vi "PXI_Host_SGL_Read_OldMethod_Benchmark.vi"() -> ()   [LabVIEW 2018]
uses:
  <vilib>/Platform/TimedLoop/XDataNode/timing_clust.ctl
  <vilib>/Platform/TimedLoop/XDataNode/nitl_modes.ctl
  <vilib>/Platform/TimedLoop/XDataNode/wakeup.ctl
  <vilib>/addons/FPGA Advanced Session Resources/LVFPGA Adv Session Resources/OpenByNameSubVI.vi
  <vilib>/rvi/interface/common/dynamic/niFpgaEscapeDelimiterAndNull.vi
  <vilib>/Utility/error.llb/Error Cluster From Error Code.vi
  <vilib>/rvi/errors/niLvFpgaAdjustHostInterfaceError.vi
  <vilib>/FPGAPlugInAG/Dynamic/niLvFpga_Close_Dynamic.vi
  <vilib>/addons/FPGA Advanced Session Resources/LVFPGA Adv Session Resources/OpenByName.xnode
  <vilib>/platform/TimedLoop/XDataNode/XDataNode.xnode
  <vilib>/rvi/interface/nirviReadWriteControl/nirviReadWriteControl.xnode
  <vilib>/rvi/interface/nirviCloseFPGA/nirviCloseFPGA.xnode
  NiFpgaLv.dll
  <vilib>/rvi/interface/Simulation/niFpgaSimulationCallBeginRW.vi
  <vilib>/Platform/TimedLoop/XDataNode/XDNodeRunTimeDep.lvlib
  <vilib>/addons/FPGA Advanced Session Resources/LVFPGA Adv Session Resources/LVFPGAAdvSessionResources.lvlib
panel:
  out "Waveform Graph":dbl[](graph)
  out "Standard Dev":dbl
  out "Execution time (s)":dbl
  out "Maximum(s)":dbl
  out "Value out":sgl
  out "error out":errorcluster
  # "Recorded time"
  # "3.37551E-5"
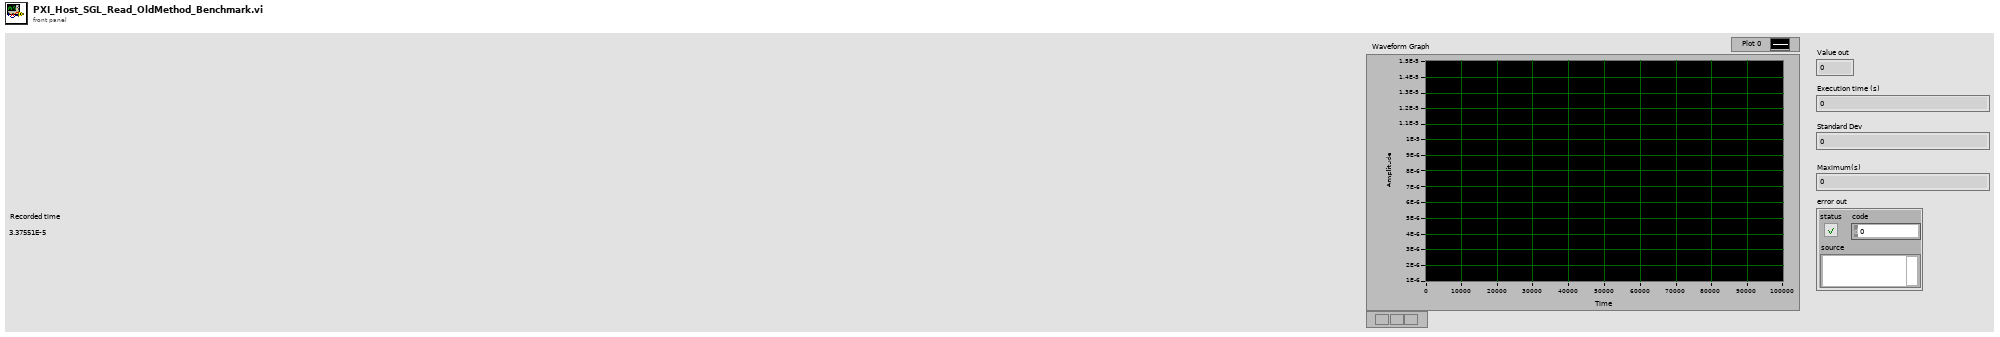
[diagram p1: front panel]
types:
  T1 = typedef "XDNodeRunTimeDep.lvlib/timing_clust.ctl" = cluster{"Expected End [f-1]":u64, "Actual End [f-1]":u64, "Finished Late? [f-1]":bool, "Expected End [i-1]":u64, "Actual End [i-1]":u64, "Finished Late? [i-1]":bool, "Expected Start [i]":u64, "Actual Start [i]":u64, "Expected Start [f]":u64, "Actual Start [f]":u64, "Source Name":string, "Structure Name":string, "Period":i64, "Deadline":i64, "Offset":i64, "Start":i64, "Priority":i32, "Timeout":i32, "Mode":T2, "Wakeup Reason":T3, "Error":errorcluster, "Source Type":string, "Secondary Source Type":string, "Global End Time":u64, "Global Start Time":u64, "Frame Duration":u64, "Iteration Duration":u64, "Assigned CPU":i32, "I/O Scan Engine Mode":u32}
  T2 = typedef "XDNodeRunTimeDep.lvlib/nitl_modes.ctl" = enum32{"No Change", "Process missed periods, maintain original phase", "Discard missed periods, maintain original phase", "Process missed periods, ignore original phase", "Discard missed periods, ignore original phase"}
  T3 = typedef "XDNodeRunTimeDep.lvlib/wakeup.ctl" = enum32{"Normal", "Aborted", "Asynchronous wakeup", "Timing source error", "Timed loop error", "Timeout"}
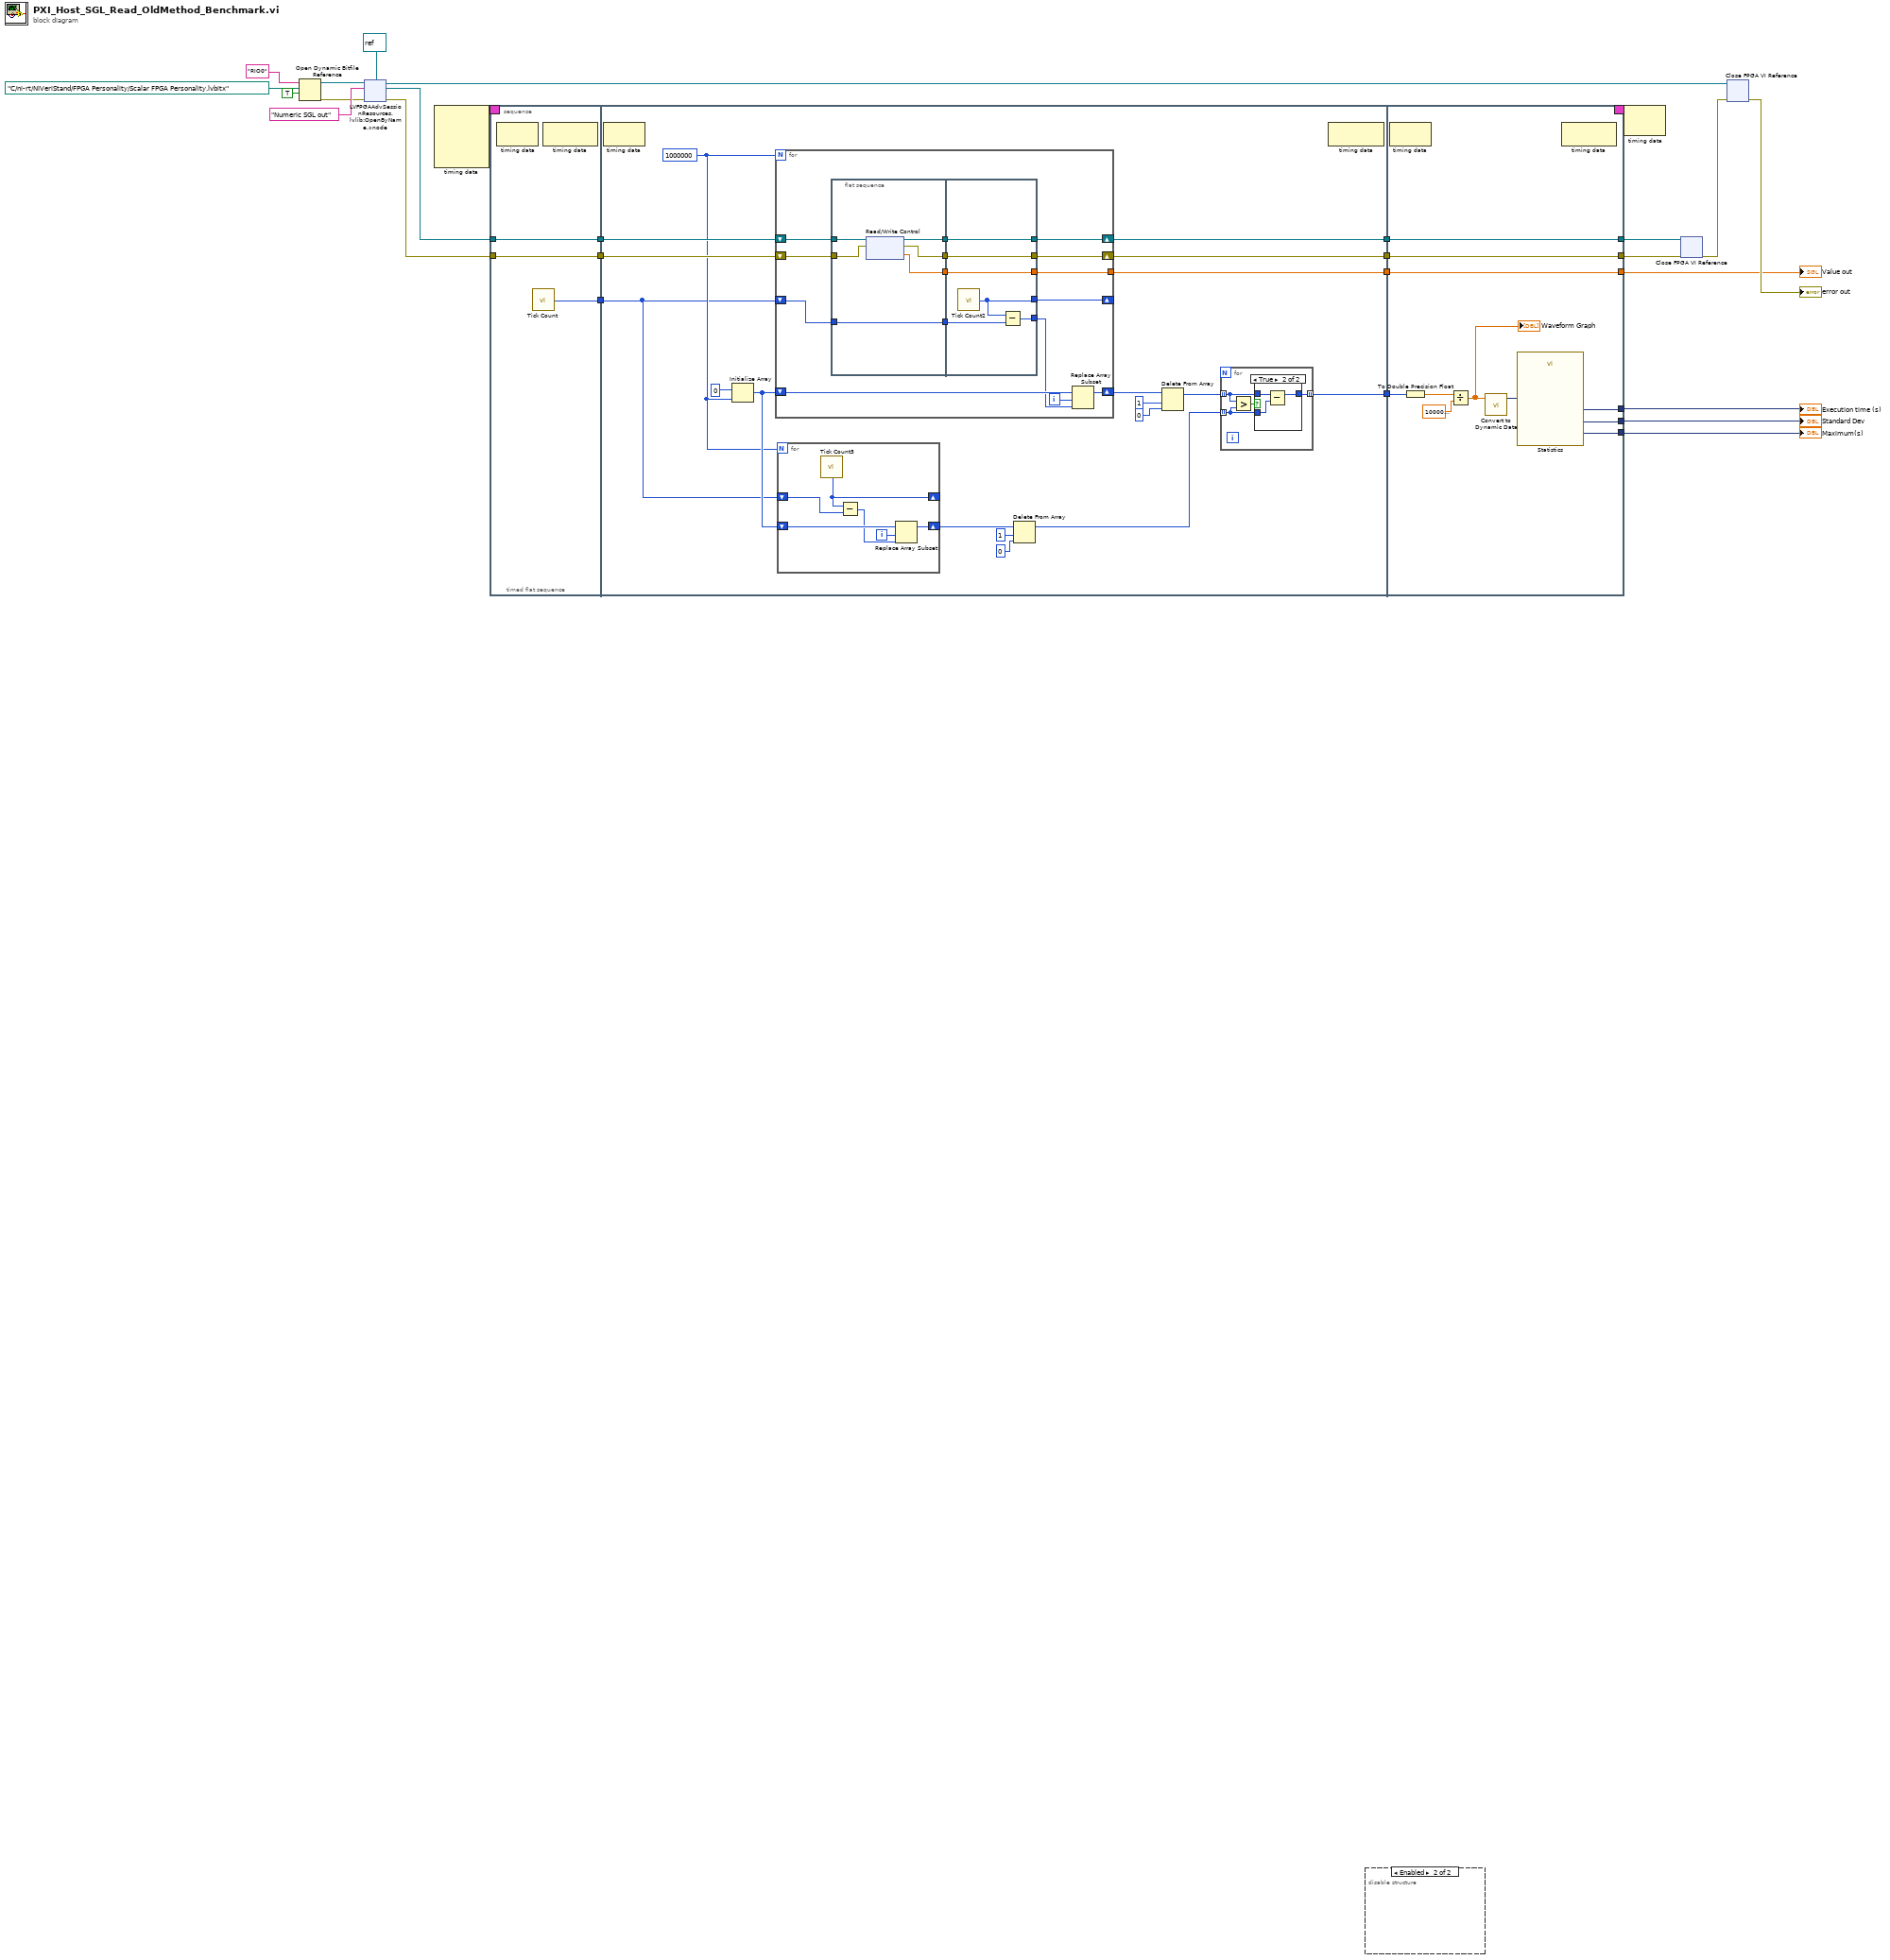
[diagram p0: block diagram]
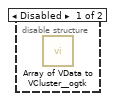
[diagram p3: hidden frame]
diagram:
  n1 = Open Dynamic Bitfile Reference(0:"RIO0" ("Device address"), 1:path "C:/ni-rt/NIVeriStand/FPGA Personality/Scalar FPGA Personality.lvbitx" ("Bitfile path"), 2:TRUE ("Run When Loaded")) -> (5:w16:refnum<k20>, 8:w14:errorcluster)  [unwired: 2 in]
  n2 = xnode "LVFPGAAdvSessionResources.lvlib:OpenByName.xnode"("FPGA VI Reference in"=w16, "Resource name in"="Numeric SGL out", "Single resource reference type in"=refnum<k20> refnum ("Type"), "Error in"=w14) -> ("Single resource reference out"=w12:refnum<k20>, "Error out"=w13:errorcluster, "FPGA VI Reference out"=w8:refnum<k20>)
  n3 = node-c288() -> (w5:T1)  [unwired: 4 in]
  n4 = timed-sequence {
    timing: w5 -> [_]
    timing-out: [_] -> w4
    tunnel: [w35] -> w17
    tunnel: w13 -> [w34]
    tunnel: w12 -> [w33]
    tunnel: [w32] -> w10
    tunnel: [w31] -> w6
    tunnel: [w23] -> w3
    tunnel: [w22] -> w2
    tunnel: [w21] -> w1
    n5 = timed-flat-sequence {
      tunnel: w33 -> [w37]
      tunnel: w34 -> [w38]
      tunnel: [w38] -> w30
      tunnel: [w37] -> w29
      tunnel: [w36] -> w28
      tunnel: w30 -> [w57]
      tunnel: w29 -> [w56]
      tunnel: w28 -> [w41]
      tunnel: [w58] -> w27
      tunnel: [w55] -> w26
      tunnel: [w54] -> w25
      tunnel: [w42] -> w24
      tunnel: [w110] -> w31
      tunnel: [w111] -> w32
      tunnel: [w112] -> w35
      tunnel: w27 -> [w112]
      tunnel: w26 -> [w111]
      tunnel: w25 -> [w110]
      tunnel: w24 -> [w105]
      tunnel: [w104] -> w23
      tunnel: [w103] -> w22
      tunnel: [w102] -> w21
      frame #0 {
        n6 = node-c288() -> ()  [unwired: 1 in, 1 out]
        n7 = call "Tick Count"() -> ("Tick Count(Ticks)"=w36:u32)
        n8 = node-c288() -> ()  [unwired: 1 in, 1 out]
      }
      frame #1 {
        w43 = 1000000
        n9 = node-c288() -> ()  [unwired: 1 in, 1 out]
        n10 = Initialize Array(u32 0 ("Tick Count(uSec)"), w43) -> (w44:u32[])
        n11 = for {
          N: w43 -> [_]
          tunnel: [w76] -> w54
          shift-right: [w80] -> w58
          shift-left: w57 -> [w79]
          shift-right: [w77] -> w55
          shift-left: w56 -> [w78]
          shift-right: [w73] -> _
          shift-left: w41 -> [w75]
          shift-right: [w69] -> w46
          shift-left: w44 -> [w72]
          i -> [w70]
          n12 = flat-sequence {
            tunnel: [w87] -> w83
            tunnel: [w86] -> w82
            tunnel: [w85] -> w81
            tunnel: w78 -> [w89]
            tunnel: w79 -> [w88]
            tunnel: w75 -> [w84]
            tunnel: [w84] -> w74
            tunnel: [w95] -> w71
            tunnel: w83 -> [w94]
            tunnel: [w94] -> w80
            tunnel: [w93] -> w76
            tunnel: w82 -> [w93]
            tunnel: w81 -> [w92]
            tunnel: [w92] -> w77
            tunnel: w74 -> [w91]
            tunnel: [w90] -> w73
            frame #0 {
              n13 = xnode "Read/Write Control"("FPGA VI Reference In"=w89, "error in"=w88) -> ("FPGA VI Reference Out"=w85:refnum<k20>, "error out"=w87:errorcluster, "Value"=w86:sgl)
            }
            frame #1 {
              n14 = call "Tick Count2"() -> ("Tick Count(Ticks)"=w90:u32)
              n15 = Subtract(x=w90, y=w91) -> (x-y=w95:u32)
            }
          }
          n16 = Replace Array Subset(array=w72, new element=w71, index=w70) -> (w69:u32[])
        }
        n17 = for {
          N: w43 -> [_]
          shift-right: [w96] -> w50
          shift-left: w44 -> [w99]
          shift-right: [w101] -> _
          shift-left: w41 -> [w100]
          i -> [w97]
          n18 = call "Tick Count3"() -> ("Tick Count(Ticks)"=w101:u32)
          n19 = Subtract(x=w101, y=w100) -> (x-y=w98:u32)
          n20 = Replace Array Subset(array=w99, new element=w98, index=w97) -> (w96:u32[])
        }
        n21 = Delete From Array(array=w50, length=1, index=0) -> (array with subset deleted=w45:u32[])  [unwired: 1 out]
        n22 = Delete From Array(array=w46, length=1, index=0) -> (array with subset deleted=w47:u32[])  [unwired: 1 out]
        n23 = for {
          tunnel: [w62] -> w42 mode=indexing
          tunnel: w47 -> [w61] mode=indexing
          tunnel: w45 -> [w60] mode=indexing
          n24 = Greater?(x=w61, y=w60) -> (0:w59:bool)
          n25 = case shown="True" w59 {
            tunnel: w61 -> [w63 w66]
            tunnel: w60 -> [_ w65]
            tunnel: [w63 w64] -> w62
            frame False {
            }
            frame True {
              n26 = Subtract(x=w66, y=w65) -> (x-y=w64:u32)
            }
          }
        }
        n27 = node-c288() -> ()  [unwired: 1 in, 1 out]
      }
      frame #2 {
        n28 = node-c288() -> ()  [unwired: 1 in, 1 out]
        n29 = To Double Precision Float(number=w105) -> (double precision float=w109:dbl[])
        n30 = Divide(x=w109, y=1000000000.0) -> (x/y=w106:dbl[])
        "Waveform Graph" <- w106
        n31 = call "Convert to Dynamic Data"("Array"=w106) -> ("Dynamic Data Type"=w107:dynamicdata)  [unwired: 3 in]
        n32 = call "Statistics"("Signals"=w107) -> ("Standard Dev"=w103:dynamicdata, "Arithmetic Mean"=w104:dynamicdata, "Maximum"=w102:dynamicdata)  [unwired: 23 in, 1 out]
        n33 = node-c288() -> ()  [unwired: 1 in, 1 out]
      }
    }
  }
  "Value out" <- w6
  "Maximum(s)" <- w1
  "Execution time (s)" <- w3
  "Standard Dev" <- w2
  n34 = disable-structure shown="Enabled" {
    frame Disabled {
      n35 = call <userlib>:"Array of VData to VCluster__ogtk.vi"() -> ()  [unwired: 10 in, 2 out]
    }
    frame Enabled {
    }
  }
  n36 = node-c288(w4) -> ()  [unwired: 1 out]
  n37 = xnode "Close FPGA VI Reference"("FPGA VI Reference In"=w10, "error in"=w17) -> ("error out"=w9:errorcluster)
  n38 = xnode "Close FPGA VI Reference"("FPGA VI Reference In"=w8, "error in"=w9) -> ("error out"=→"error out":errorcluster)
